vi "Read_TDL_BRAM_data.vi"(7 "error in":errorcluster, 10 "VISA  in":refnum<visa-resource-name>) -> (0 "error out":errorcluster, 2 "RdReg Data":u8[](array[numeric]), 3 "VISA out":refnum<visa-resource-name>)   [LabVIEW 2019]
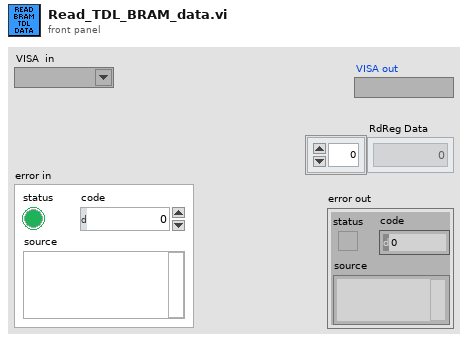
[diagram p1: front panel]
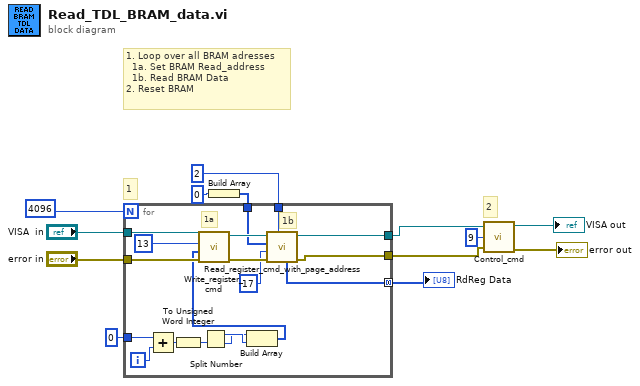
[diagram p0: block diagram]
diagram:
  # "1"
  # "2"
  # "1. Loop over all BRAM adresses\n  1a. Set BRAM Read_address\n  1b. Read BRAM Data\n2. Reset BRAM"
  n1 = Build Array(u8 0 ("element")) -> (w11:u8[])
  n2 = for {
    N: 4096 -> [_]
    tunnel: "VISA  in" -> [w31]
    tunnel: "error in" -> [w30]
    tunnel: u8 2 ("y") -> [w27]
    tunnel: u8 0 -> [w24]
    tunnel: w11 -> [w18]
    tunnel: [w17] -> w9 mode=concatenating
    tunnel: [w16] -> w6
    tunnel: [w15] -> w5
    i -> [w25]
    # "1b"
    # "1a"
    n3 = Add(x=w24, y=w25) -> (x+y=w23:i32)
    n4 = To Unsigned Word Integer(number=w23) -> (unsigned 16bit integer=w20:u16)
    n5 = Split Number(x=w20) -> (hi(x)=w22:u8, lo(x)=w21:u8)
    n6 = Build Array(w21, w22) -> (w19:u8[])
    n7 = call "Write_register_cmd.vi"("Arty-7 Error In"=w30, "Data Array"=w19, "WrReg Addr"=u8 13, "Arty-7 VISA In"=w31) -> ("Arty-7 Error out"=w28:errorcluster, "Arty-7 VISA out"=w29:refnum<visa-resource-name>)  [unwired: 4 in, 2 out]
    n8 = call "Read_register_cmd_with_page_address.vi"("Words_to_read"=w27, "error in (no error)"=w28, "Register Address"=u8 17, "Page address"=w18, "VISA Refnum in"=w29) -> ("error out"=w15:errorcluster, "VISA Refnum out"=w16:refnum<visa-resource-name>, "RdReg Data"=w17:u8[])  [unwired: 4 in]
  }
  "RdReg Data" <- w9
  n9 = call "Control_cmd.vi"("Arty-7 Error In"=w5, "Control Command"=u8 9, "Arty-7 VISA In"=w6) -> ("Arty-7 Error out"=→"error out":errorcluster, "Arty-7 VISA out"=→"VISA out":refnum<visa-resource-name>)  [unwired: 2 in, 2 out]
